vi "APS read a output value.vi"(8 "error in (no error)":errorcluster caption="错误输入（无错误）", 9 "Convert_Data":dbl, 10 "Channel_No":i32, 11 "Board_ID":i32) -> (0 "error out":errorcluster caption="错误输出", 1 "Convert_Data out":dbl, 3 "function return":i32)   [LabVIEW 2011, in "APS168.lvlib"]
doc: "I32 FNTYPE APS_read_a_output_value(I32 Board_ID, I32 Channel_No, F64 *Convert_Data);"
uses:
  APS168.lvlib
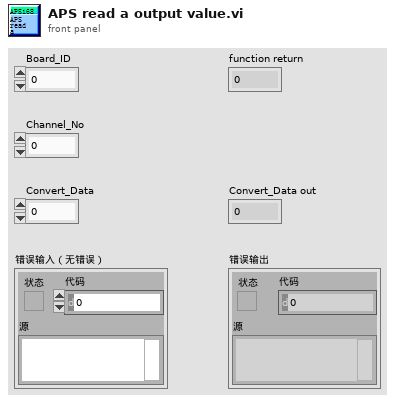
[diagram p1: front panel]
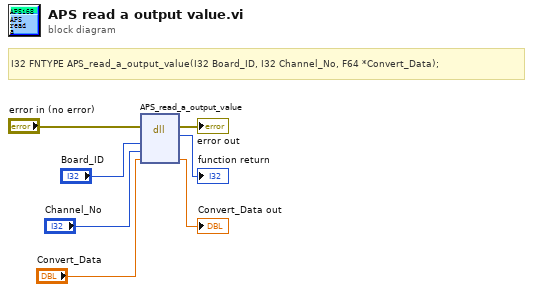
[diagram p0: block diagram]
diagram:
  # "I32 FNTYPE APS_read_a_output_value(I32 Board_ID, I32 Channel_No, F64 *Convert_Data);"
  n1 = dll-call lib="PTH1Labs E软件ADLINK 204CAPS_1_7_1_LIB line 连续运动204APS168.*" fn="APS_read_a_output_value"(error in="error in (no error)", "Board_ID"="Board_ID", "Channel_No"="Channel_No", "Convert_Data"="Convert_Data") -> (error out=→"error out":errorcluster, →"function return":i32, "Convert_Data"=→"Convert_Data out":dbl)  [unwired: 4 in, 1 out]
